vi "scratch_pad.vi"   [LabVIEW 2013]
uses:
  <instrlib>/Mercury iXX/Mercury iXX.lvlib
  <instrlib>/Mercury iXX/Public/Libraries/Control Loop/Configuration/Set/Sweep Mode (Set).vi
  <instrlib>/Mercury iXX/Public/Libraries/Control Loop.lvlib
  <instrlib>/Mercury iXX/Public/Libraries/Control Loop/Configuration/Set/Temperature Setpoint (Set).vi
  <instrlib>/Mercury iXX/Private/Controls/Command Verbs.ctl
  <instrlib>/Mercury iXX/Public/Controls/Comms Transport Layer.ctl
  <instrlib>/Mercury iXX/Private/Controls/Query Dynamic Reference.ctl
  <instrlib>/Mercury iXX/Public/Controls/Mercury Reference.ctl
types:
  T1 = typedef "Mercury iXX.lvlib/Mercury Reference.ctl" = cluster{"Comms":refnum<visa-resource-name>, "Device ID":string[], "Comms Layer":T2, "Command":string, "Query reference":T3}
  T2 = typedef "Mercury iXX.lvlib/Comms Transport Layer.ctl" = enum16{"Ethernet TCP/IP", "USB", "ISOBus - RS-232", "GPIB"}
  T3 = typedef "Mercury iXX.lvlib/Query Dynamic Reference.ctl" = refnum<vi>
  T4 = typedef "Mercury iXX.lvlib/Command Verbs.ctl" = string
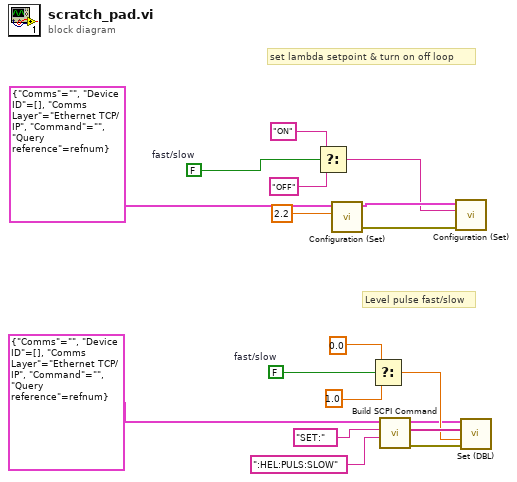
[diagram p0: block diagram]
diagram:
  w3 = FALSE  # fast/slow
  w4 = FALSE  # fast/slow
  # "set lambda setpoint & turn on off loop"
  # "Level pulse fast/slow"
  n1 = Select(t="ON" ("Sweep Mode"), s=w4, f="OFF" ("Sweep Mode")) -> (s? t:f=w15:string)
  n2 = call-poly <instrlib>:"Configuration (Set).vi"("Temperature setpoint"=2.2, "Mercury Reference In"=T1 {"Comms"="", "Device ID"=[], "Comms Layer"=enum."Ethernet TCP/IP", "Command"="", "Query reference"=refnum}) -> ("error out"=w16:errorcluster, "Mercury Reference Out"=w17:T1)  [unwired: 6 in, 2 out]
  n3 = Select(t=0.0 ("Temperature setpoint"), s=w3, f=1.0 ("Temperature setpoint")) -> (s? t:f=w9:dbl)
  n4 = call <instrlib>:"Build SCPI Command.vi"("Noun(s)"=":HEL:PULS:SLOW", "Verb"=T4 "SET:", "Mercury Reference In"=T1 {"Comms"="", "Device ID"=[], "Comms Layer"=enum."Ethernet TCP/IP", "Command"="", "Query reference"=refnum}) -> ("error out"=w6:errorcluster, "SCPI Message(s)"=w12:string[], "Mercury Reference Out"=w5:T1)  [unwired: 6 in]
  n5 = call-poly <instrlib>:"Configuration (Set).vi"("error in"=w16, "Sweep Mode"=w15, "Mercury Reference In"=w17) -> ()  [unwired: 5 in, 4 out]
  n6 = call <instrlib>:"Set (DBL).vi"("error in"=w6, "Command Value (Dbl)"=w9, "SCPI Message(s)"=w12, "Mercury Reference In"=w5) -> ()  [unwired: 4 in, 4 out]
